vi "report read.vi"(0 "connection reference":T2, 1 "table":string="Reportgen", 4 "DB write":T1, 5 "error in (no error)":errorcluster, 7 "Enter Part Unique id":string="A1234567B567", 8 "search dataString":string, 11 "Enum":enum16{"Write", "Read"}(ring)=enum."Read") -> (12 "Search Reverse":string[][](table), 14 "connection reference out":T2, 15 "last id":variant[][](array[variant]), 16 "Search result":string[][](table), 17 "DMC TESTED:T":bool, 19 "error out":errorcluster)   [LabVIEW 2023]
uses:
  <vilib>/addons/database/Connection.llb/Conn ObjectReference.ctl
  <vilib>/addons/database/_DB Variant To Data/Database Variant To Data.xnode
  <vilib>/addons/database/NI_Database_API.lvlib
panel:
  out "data":string[][](array[string])
  out "columns":string[](array[string])
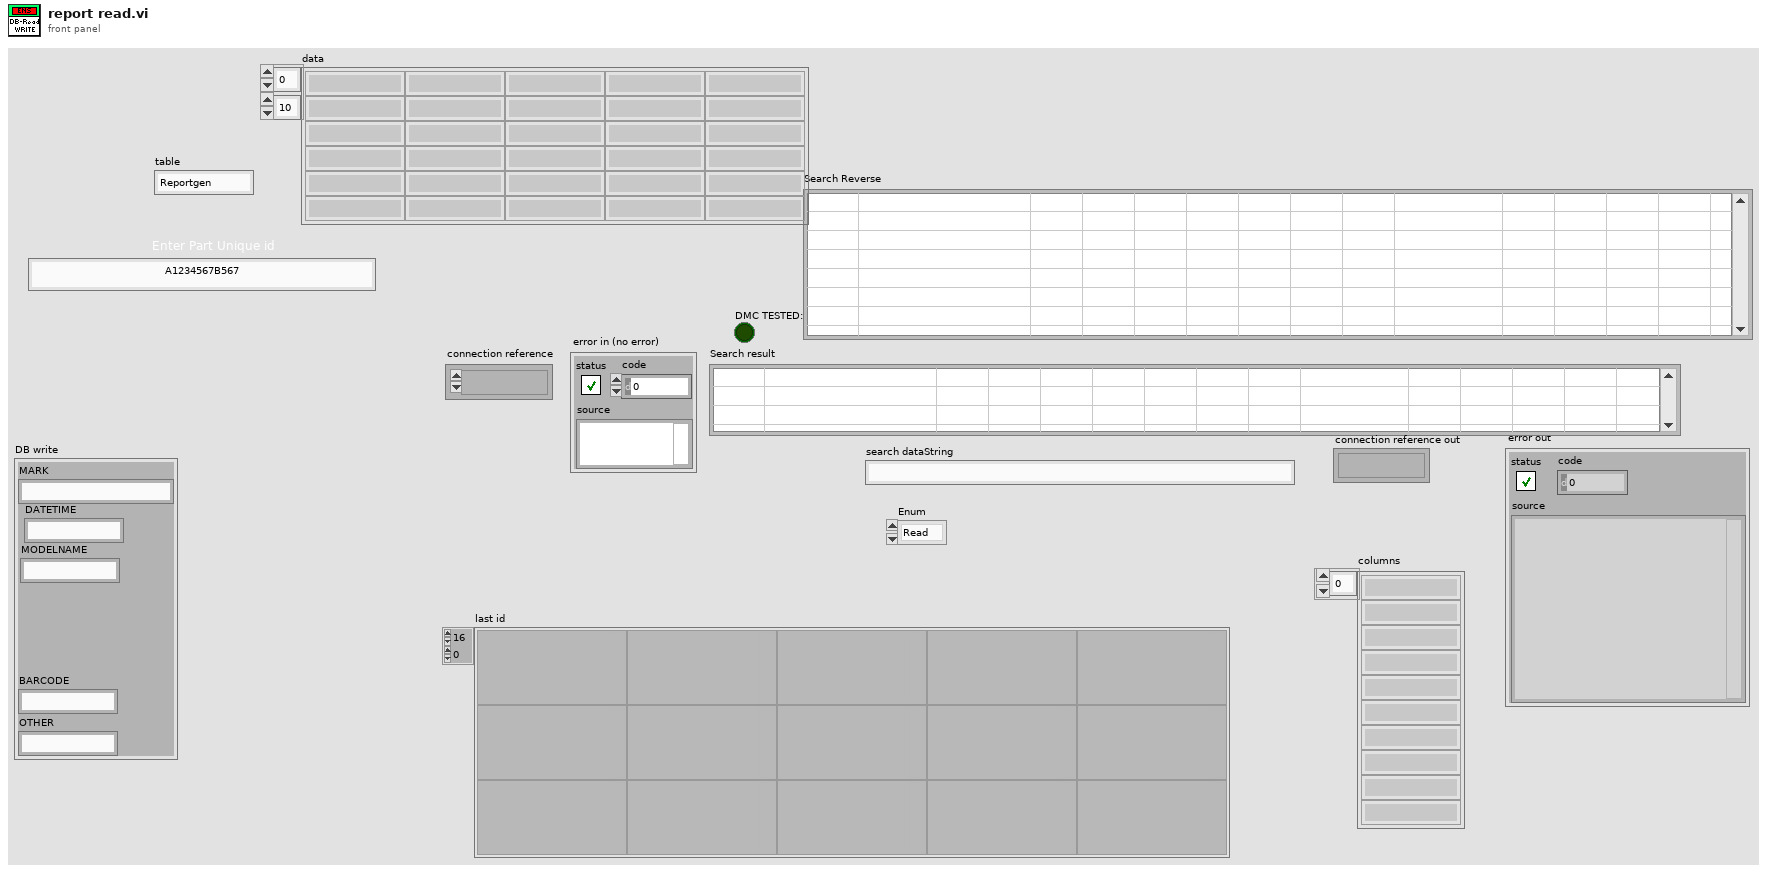
[diagram p1: front panel]
types:
  T1 = cluster{"DATETIME":string, "MODELNAME":string, "BARCODE":string, "MARK":string, "OTHER":string}
  T2 = typedef "NI_Database_API.lvlib/Conn ObjectReference.ctl" = refnum<k1>
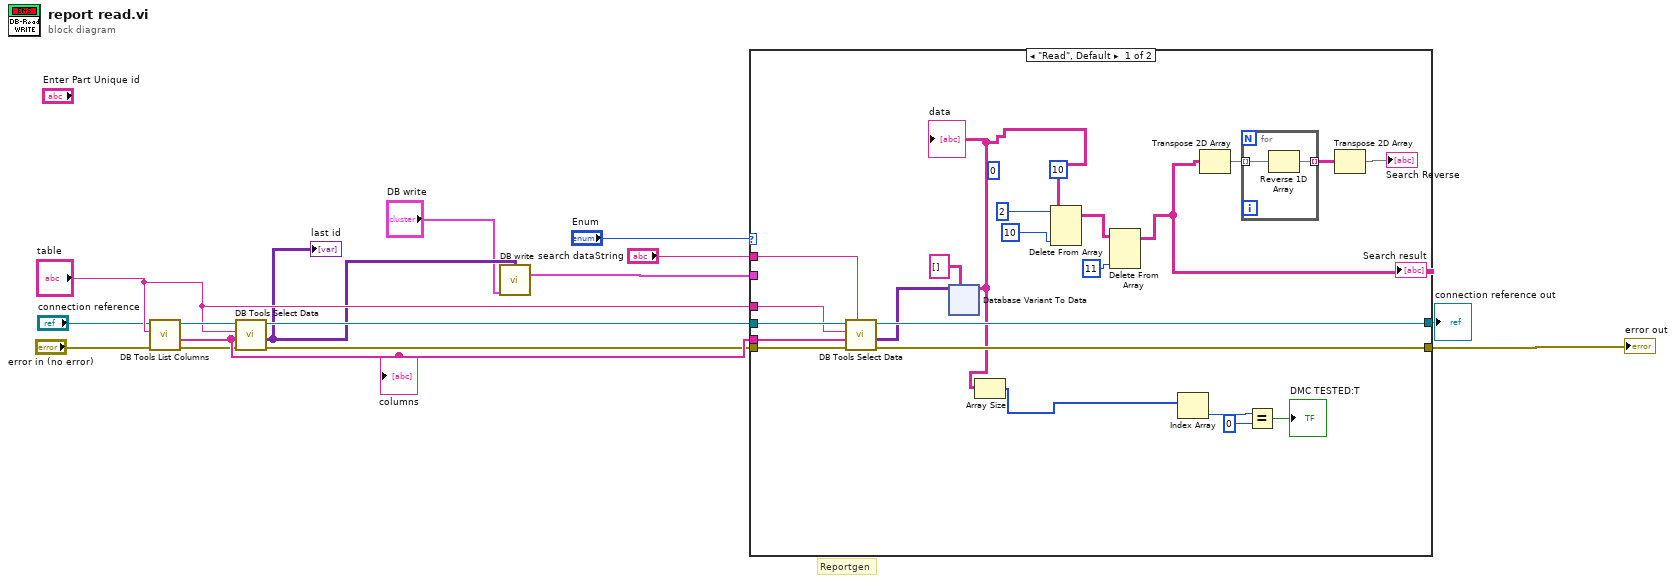
[diagram p0: block diagram]
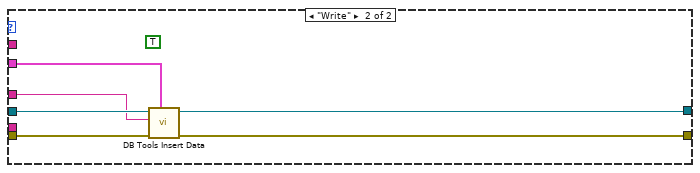
[diagram p2: hidden frame]
diagram:
  # "Reportgen"
  n1 = call <vilib>:"DB Tools List Columns.vi"("error in (no error)"="error in (no error)", "table"="table", "connection reference"="connection reference") -> ("error out"=w13:errorcluster, "columns"=w15:string[], "connection reference out"=w14:T2)  [unwired: 1 in, 1 out]
  "columns" <- w15
  n2 = call <vilib>:"DB Tools Select Data.vi"("error in (no error)"=w13, "columns"=w15, "table"="table", "connection reference"=w14) -> ("error out"=w12:errorcluster, "data"=w3:variant[][], "connection reference out"=w11:T2)  [unwired: 2 in]
  "last id" <- w3
  n3 = call "DB write.vi"("DB data"=w3, "DB write"="DB write") -> ("DB write"=w2:T1)  [unwired: 13 in]
  n4 = case shown="\"Read\", Default" "Enum" {
    tunnel: [w33 w89] -> w4
    tunnel: [w32 w88] -> w5
    tunnel: w15 -> [w34 _]
    tunnel: w12 -> [w36 w87]
    tunnel: w11 -> [w37 w86]
    tunnel: "table" -> [w35 w84]
    tunnel: w2 -> [_ w85]
    tunnel: "search dataString" -> [w31 _]
    frame "Read", Default {
      (unwired) 10 ("disabled index (col)")
      (unwired) 0 ("disabled index (col)")
      n5 = call <vilib>:"DB Tools Select Data.vi"("condition"=w31, "error in (no error)"=w36, "columns"=w34, "table"=w35, "connection reference"=w37) -> ("error out"=w32:errorcluster, "data"=w29:variant[][], "connection reference out"=w33:T2)  [unwired: 1 in]
      n6 = xnode "Database Variant To Data"("database variant"=w29, "type"=string[][] [] ("Array")) -> ("data"=w21:string[][])  [unwired: 1 in, 1 out]
      "data" <- w21
      n7 = Array Size(array=w21) -> (size(s)=w28:i32[])
      n8 = Delete From Array(array=w21, length=2, index (col)=10 ("index (row)")) -> (array with subset deleted=w18:string[][])  [unwired: 1 in, 1 out]
      n9 = Delete From Array(array=w18, index (col)=11 ("length")) -> (array with subset deleted=w17:string[][])  [unwired: 2 in, 1 out]
      "Search result" <- w17
      n10 = Index Array(array=w28) -> (element=w27:i32)  [unwired: 1 in]
      n11 = Transpose 2D Array(2D array=w17) -> (transposed array=w24:string[][])
      n12 = for {
        tunnel: w24 -> [w39] mode=indexing
        tunnel: [w38] -> w23 mode=indexing
        n13 = Reverse 1D Array(array=w39) -> (reversed array=w38:string[])
      }
      n14 = Equal?(x=w27, y=0) -> (x = y?=→"DMC TESTED:T":bool)
      n15 = Transpose 2D Array(2D array=w23) -> (transposed array=→"Search Reverse":string[][])
    }
    frame "Write" {
      (unwired) TRUE ("create table? (F)")
      n16 = call <vilib>:"DB Tools Insert Data.vi"("data"=w85, "error in (no error)"=w87, "table"=w84, "connection reference"=w86) -> ("error out"=w88:errorcluster, "connection reference out"=w89:T2)  [unwired: 6 in]
    }
  }
  "error out" <- w5
  "connection reference out" <- w4
